vi "Autonomous Independent.vi"   [LabVIEW 2015]
doc: "This VI is called when autonomous begins, and will automatically be terminated when autonomous ends. You can carry out timed or sensor driven robot movement independently without needing to return to the caller."
uses:
  <vilib>/Rock Robotics/WPI/Relay/WPI_RelayValue.ctl
  <vilib>/Rock Robotics/Network Tables/SD Read String.vi
  <vilib>/Rock Robotics/WPI/Utilities/WPI_GetSetVariantRefNum.vi
  Robot Global Data.vi
  <vilib>/Rock Robotics/WPI/RobotDrive/WPI_RobotDriveMecanumDrive_Cartesian.vi
  <vilib>/addons/control/pid/pid.llb/PID (DBL).vi
  <vilib>/Rock Robotics/Network Tables/SD Write Numeric Array.vi
  SimpleGyro/SimpleGyro.lvlib
  <vilib>/addons/control/pid/NI_PID_pid.lvlib
panel:
  # "Be sure to right-click and choose Data Operations>>Make Current Value default if you want to save the array values with the VI"
types:
  T1 = typedef "WPI_RelayValue.ctl" = enum16{"Off", "On", "Forward", "Reverse"}
  T2 = cluster{"proportional gain (Kc)":dbl, "integral time (Ti, min)":dbl, "derivative time (Td, min)":dbl}
  T3 = typedef "SimpleGyro.lvlib/WPI_SimpleGyroDevRef.ctl" = cluster{"DevStatus":errorcluster, "Handle":i32, "SPI Bus":T4, "Device Found":bool, "Sample Rate":dbl}
  T4 = typedef "spi_bus.ctl" = enum16{"SPI On-Board, CS0", "SPI On-Board, CS1", "SPI On-Board, CS2", "SPI On-Board, CS3", "SPI MXP", "Invalid"}
  T5 = typedef "WPI_RobotDriveDevRef.ctl" = cluster{"DevStatus":errorcluster, "Motors[]":T6[], "Square Inputs":bool, "Max Output":dbl}
  T6 = typedef "WPI_MotorControlDeviceRef.ctl" = cluster{"DeviceStatus":errorcluster, "Type":T7, "PWM":cluster{"PWM Channel":T8, "DeadBand":T9}, "CAN":cluster{"Device Number":u8, "Control Mode":T10, "Semaphore":T11, "Max Vout":dbl, "TalonSRX Control Mode":T12}, "Invert":bool, "TransformRef":T13, "InvTransformRef":T13}
  T7 = typedef "WPI_MotorControlType.ctl" = enum16{"PWM", "CAN", "CANTalonSRX"}
  T8 = typedef "FPGA_DIOPWMChannel.ctl" = enum8{"PWM 0", "PWM 1", "PWM 2", "PWM 3", "PWM 4", "PWM 5", "PWM 6", "PWM 7", "PWM 8", "PWM 9", "PWM MXP 0", "PWM MXP 1", "PWM MXP 2", "PWM MXP 3", "PWM MXP 4", "PWM MXP 5", "PWM MXP 6", "PWM MXP 7", "PWM MXP 8", "PWM MXP 9", "Invalid"}
  T9 = typedef "WPI_PWMDeadband.ctl" = cluster{"Name":string, "maxPositivePwm":i32, "minPositivePwm":i32, "centerPwm":i32, "maxNegativePwm":i32, "minNegativePwm":i32, "angularRange":u16}
  T10 = typedef "WPI_CANJaguar_ControlMode.ctl" = enum8{"Percent VBus", "Current", "Speed", "Position", "Voltage"}
  T11 = typedef "Semaphore RefNum" = refnum<k1>
  T12 = typedef "WPI_CANTalonSRX_APIControlMode.ctl" = enum8{"Percent VBus", "Speed", "Position", "Slave", "Unchanged / Invalid"}
  T13 = typedef "WPI_PWMTransform_ConPane.ctl" = refnum<vi>
  T14 = typedef "WPI_EncoderDevRef.ctl" = cluster{"DevStatus":errorcluster, "EncoderIndex":T15, "CounterIndex":T16, "DistancePerCount":dbl, "Decoding Type":T17}
  T15 = typedef "FPGA_EncoderIdx.ctl" = enum8{"Enc 0", "Enc 1", "Enc 2", "Enc 3", "Enc 4", "Enc 5", "Enc 6", "Enc 7", "Invalid"}
  T16 = typedef "FPGA_CounterCtrSystemIndex.ctl" = enum8{"Ctr 0", "Ctr 1", "Ctr 2", "Ctr 3", "Ctr 4", "Ctr 5", "Ctr 6", "Ctr 7", "Invalid"}
  T17 = typedef "WPI_EncoderType.ctl" = enum16{"1x", "2x", "4x"}
  T18 = typedef "WPI_RelayDevRef.ctl" = cluster{"DevStatus":errorcluster, "Relay Channel":T19, "Relay Direction":T20}
  T19 = typedef "FPGA_DIORelayChannel.ctl" = enum8{"Relay 0", "Relay 1", "Relay 2", "Relay 3", "Invalid"}
  T20 = typedef "WPI_RelayDirection.ctl" = enum16{"Both directions", "Forward only", "Reverse only"}
  T21 = cluster{"SimpleGyroDevRef":T3, "RobotDriveDevRef":T5, "EncoderDevRef":T14, "MotorControlDevRef":T6, "RelayDevRef":T18}
  T22 = cluster{"SimpleGyroDevRef":T3, "RobotDriveDevRef":T5, "EncoderDevRef":T14, "MotorControlDevRef":T6, "RelayDevRef":T18, "MotorControlDevRef":T6}
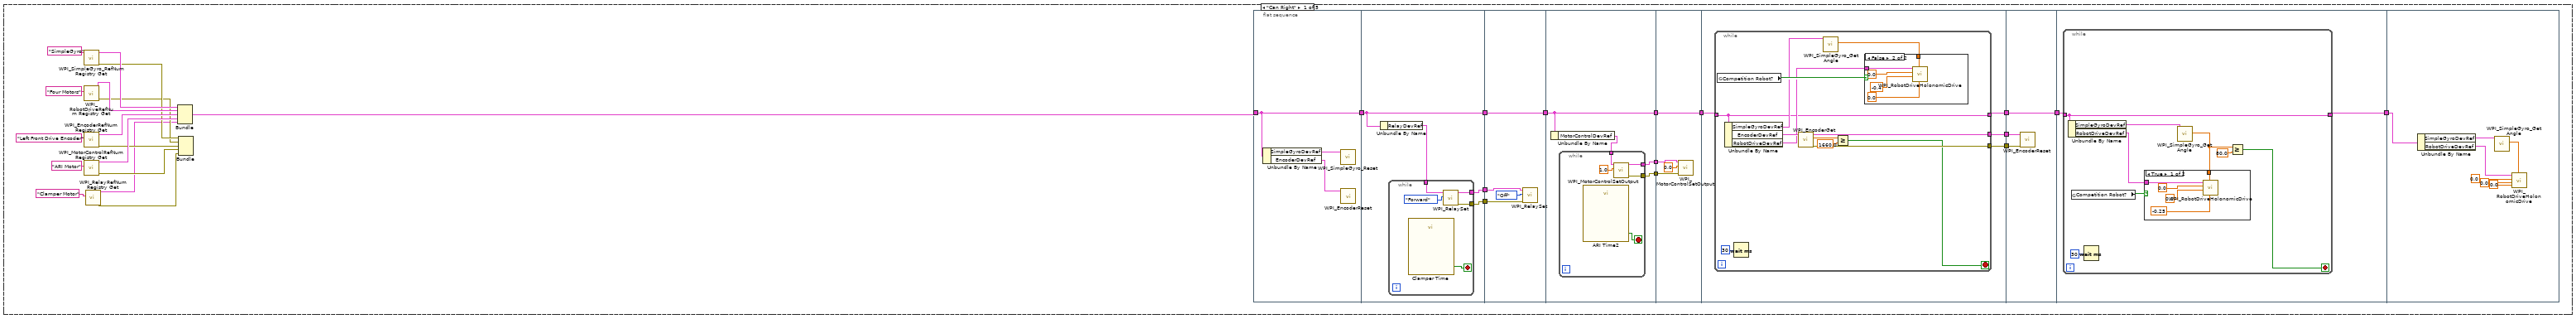
[diagram p2: hidden frame]
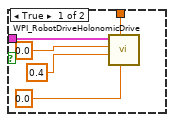
[diagram p3: hidden frame]
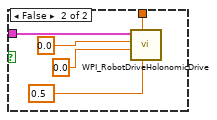
[diagram p4: hidden frame]
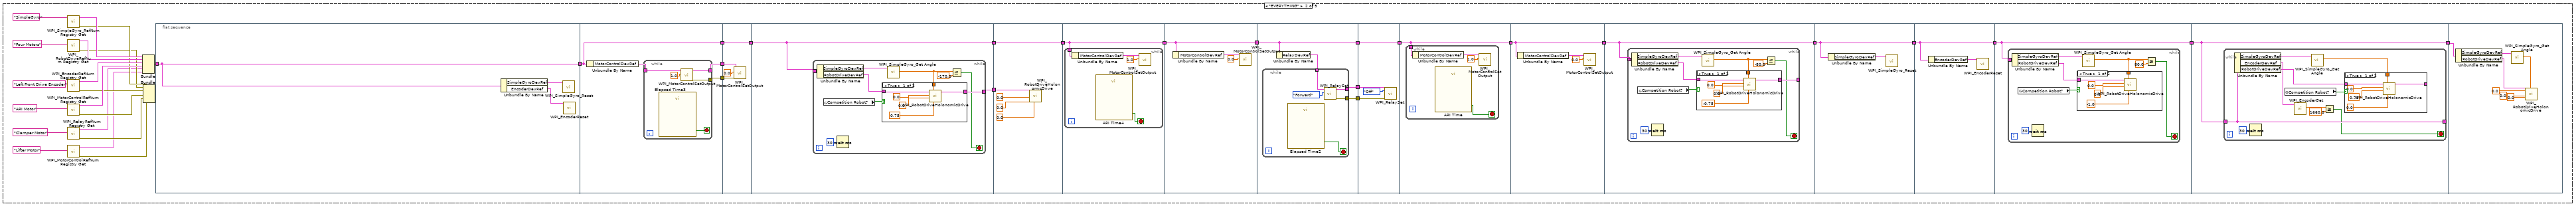
[diagram p5: hidden frame]
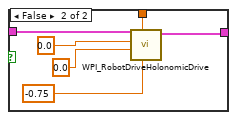
[diagram p6: hidden frame]
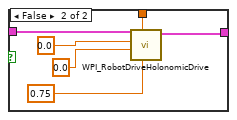
[diagram p7: hidden frame]
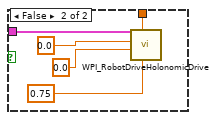
[diagram p8: hidden frame]
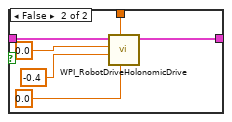
[diagram p9: hidden frame]
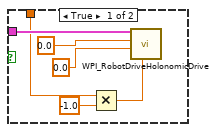
[diagram p10: hidden frame]
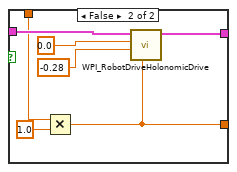
[diagram p11: hidden frame]
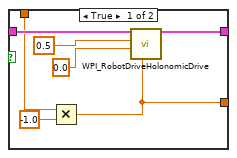
[diagram p12: hidden frame]
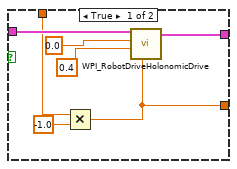
[diagram p13: hidden frame]
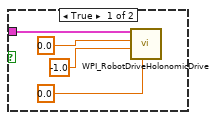
[diagram p14: hidden frame]
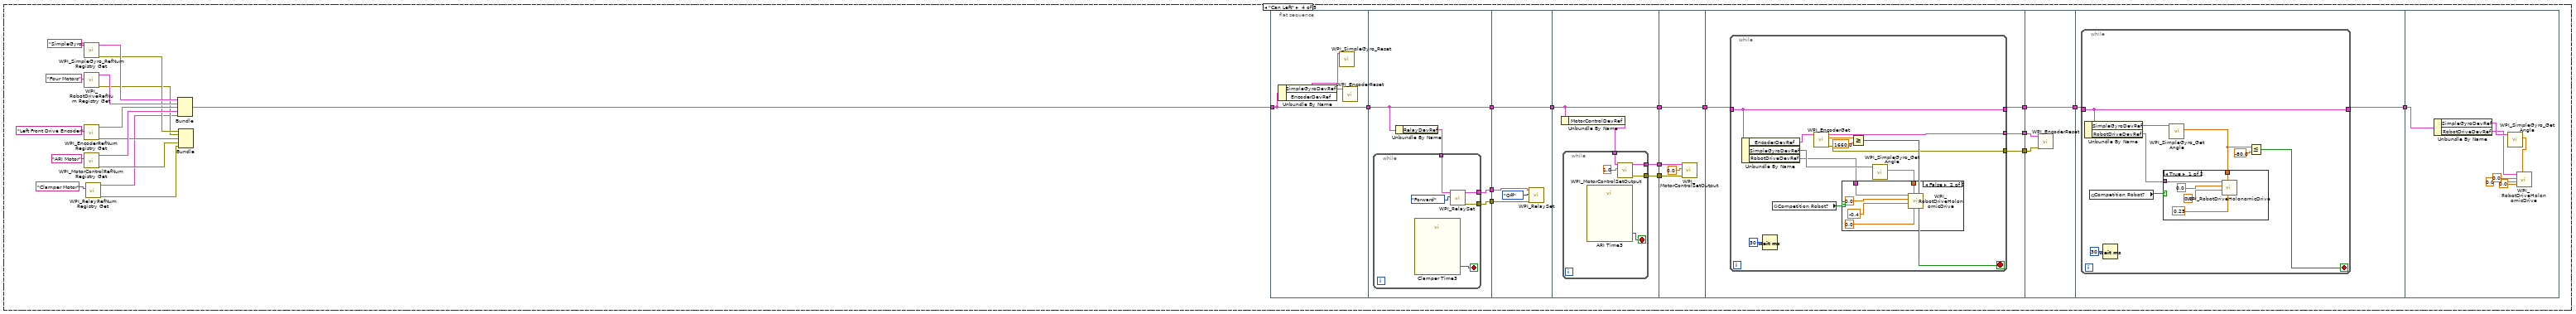
[diagram p15: hidden frame]
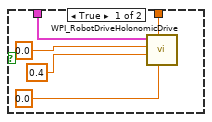
[diagram p16: hidden frame]
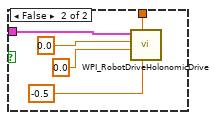
[diagram p17: hidden frame]
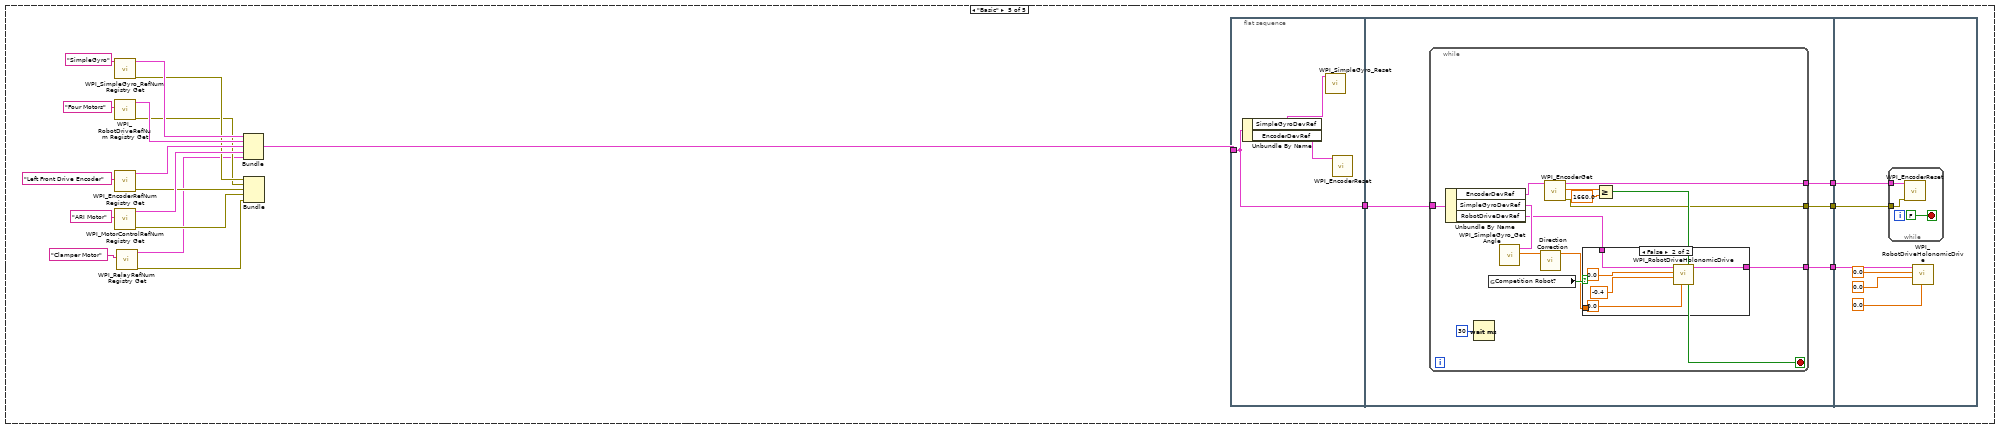
[diagram p18: hidden frame]
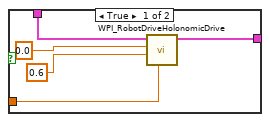
[diagram p19: hidden frame]
diagram:
  # "Every 20ms, report that we are running autonomous\ncode. Loop will abort the same time as the VI."
  n1 = call-poly <vilib>:"SD Read Value.vi"("Name"="AUTO") -> ("String"=w2:string)  [unwired: 8 in, 2 out]
  n2 = case shown="\"Totes Totes\", Default" w2 {
    frame "Can Right" {
      n3 = call "WPI_SimpleGyro_RefNum Registry Get.vi"("refnum name"="SimpleGyro") -> ("error out"=w18:errorcluster, "SimpleGyroDevRef"=w22:T3)  [unwired: 9 in]
      n4 = call <vilib>:"WPI_RobotDriveRefNum Registry Get.vi"("refnum name"="Four Motors") -> ("error out"=w17:errorcluster, "RobotDriveDevRef"=w21:T5)  [unwired: 1 in, 8 out]
      n5 = call <vilib>:"WPI_EncoderRefNum Registry Get.vi"("refnum name"="Left Front Drive Encoder") -> ("error out"=w16:errorcluster, "EncoderDevRef"=w20:T14)  [unwired: 9 in]
      n6 = call <vilib>:"WPI_MotorControlRefNum Registry Get.vi"("refnum name"="ARI Motor") -> ("error out"=w15:errorcluster, "MotorControlDevRef"=w19:T6)  [unwired: 9 in]
      n7 = call <vilib>:"WPI_RelayRefNum Registry Get.vi"("refnum name"="Clamper Motor") -> ("error out"=w10:errorcluster, "RelayDevRef"=w11:T18)  [unwired: 9 in]
      n8 = Bundle("SimpleGyroDevRef"=w22, "RobotDriveDevRef"=w21, "EncoderDevRef"=w20, "MotorControlDevRef"=w19, "RelayDevRef"=w11) -> (w14:T21)  [unwired: 1 in]
      n9 = Bundle("error out"=w18, "error out"=w17, "error out"=w16, "error out"=w15, "error out"=w10) -> ()  [unwired: 1 in, 1 out]
      n10 = flat-sequence {
        tunnel: w14 -> [w33]
        tunnel: [w33] -> w13
        tunnel: [w39] -> w32
        tunnel: [w38] -> w31
        tunnel: w13 -> [w36]
        tunnel: [w36] -> w8
        tunnel: w32 -> [w47]
        tunnel: w31 -> [w46]
        tunnel: [w45] -> w9
        tunnel: w8 -> [w45]
        tunnel: [w52] -> w30
        tunnel: [w51] -> w29
        tunnel: w9 -> [w49]
        tunnel: [w49] -> w6
        tunnel: w30 -> [w60]
        tunnel: w29 -> [w59]
        tunnel: [w58] -> w7
        tunnel: w6 -> [w58]
        tunnel: [w65] -> w28
        tunnel: [w64] -> w27
        tunnel: w7 -> [w63]
        tunnel: [w62] -> w4
        tunnel: w28 -> [w90]
        tunnel: w27 -> [w89]
        tunnel: [w88] -> w5
        tunnel: w4 -> [w88]
        tunnel: w5 -> [w92]
        tunnel: [w91] -> w3
        tunnel: w3 -> [w113]
        frame #0 {
          n11 = Unbundle By Name(w33) -> ("SimpleGyroDevRef"=w35:T3, "EncoderDevRef"=w34:T14)
          n12 = call "WPI_SimpleGyro_Reset.vi"("SimpleGyroDevRef"=w35) -> ()  [unwired: 9 in, 2 out]
          n13 = call <vilib>:"WPI_EncoderReset.vi"("EncoderDevRef"=w34) -> ()  [unwired: 9 in, 2 out]
        }
        frame #1 {
          n14 = Unbundle By Name(w36) -> ("RelayDevRef"=w37:T18)
          n15 = while {
            tunnel: [w43] -> w39
            tunnel: [w42] -> w38
            tunnel: w37 -> [w40]
            stop <- w41 stop-if-true
            n16 = call "Clamper Time"() -> ("Time has Elapsed"=w41:bool)  [unwired: 12 in, 7 out]
            n17 = call <vilib>:"WPI_RelaySet.vi"("RelayValue"=WPI_RelayValue."Forward", "RelayDevRef"=w40) -> ("error out"=w42:errorcluster, "RelayDevRef"=w43:T18)  [unwired: 8 in]
          }
        }
        frame #2 {
          n18 = call <vilib>:"WPI_RelaySet.vi"("error in (no error)"=w46, "RelayValue"=WPI_RelayValue."Off", "RelayDevRef"=w47) -> ()  [unwired: 7 in, 2 out]
        }
        frame #3 {
          n19 = Unbundle By Name(w49) -> ("MotorControlDevRef"=w50:T6)
          n20 = while {
            tunnel: [w55] -> w52
            tunnel: [w54] -> w51
            tunnel: w50 -> [w53]
            stop <- w57 stop-if-true
            n21 = call "ARI Time2"() -> ("Time has Elapsed"=w57:bool)  [unwired: 12 in, 7 out]
            n22 = call <vilib>:"WPI_MotorControlSetOutput.vi"("Output"=1.0, "MotorControlDevRef"=w53) -> ("error out"=w55:errorcluster, "MotorControlDevRef"=w54:T6)  [unwired: 7 in, 1 out]
          }
        }
        frame #4 {
          n23 = call <vilib>:"WPI_MotorControlSetOutput.vi"("error in (no error)"=w60, "Output"=0.0, "MotorControlDevRef"=w59) -> ()  [unwired: 6 in, 3 out]
        }
        frame #5 {
          n24 = while {
            tunnel: [w75] -> w65
            tunnel: [w74] -> w64
            tunnel: w63 -> [w67]
            tunnel: [w67] -> w62
            stop <- w66 stop-if-true
            n25 = global read "Robot Global Data.vi" "Competition Robot?"() -> (w72:bool)
            n26 = Unbundle By Name(w67) -> ("SimpleGyroDevRef"=w70:T3, "EncoderDevRef"=w69:T14, "RobotDriveDevRef"=w68:T5)
            n27 = Wait (ms)(milliseconds to wait=u32 30) -> ()  [unwired: 1 out]
            n28 = call <vilib>:"WPI_EncoderGet.vi"("EncoderDevRef"=w69) -> ("error out"=w74:errorcluster, "Distance"=w77:dbl, "EncoderDevRef"=w75:T14)  [unwired: 5 in, 3 out]
            n29 = call "WPI_SimpleGyro_Get Angle.vi"("SimpleGyroDevRef"=w70) -> ("Angle"=w73:dbl)  [unwired: 8 in, 2 out]
            n30 = Greater Or Equal?(x=w77, y=1660.0) -> (x >= y?=w66:bool)
            n31 = case shown="False" w72 {
              tunnel: w73 -> [w79 w84]
              tunnel: w68 -> [w78 w83]
              frame True {
                n32 = call-poly <vilib>:"WPI_RobotDriveHolonomicDrive.vi"("Rotation"=0.0, "Gyro Angle"=w79, "Y"=0.4 ("X axis value"), "X"=0.0 ("X axis value"), "RobotDriveDevRef"=w78) -> ()  [unwired: 4 in, 3 out]
              }
              frame False {
                n33 = call-poly <vilib>:"WPI_RobotDriveHolonomicDrive.vi"("Rotation"=0.0, "Gyro Angle"=w84, "Y"=-0.4 ("X axis value"), "X"=0.0 ("X axis value"), "RobotDriveDevRef"=w83) -> ()  [unwired: 4 in, 3 out]
              }
            }
          }
        }
        frame #6 {
          n34 = call <vilib>:"WPI_EncoderReset.vi"("error in (no error)"=w89, "EncoderDevRef"=w90) -> ()  [unwired: 8 in, 2 out]
        }
        frame #7 {
          n35 = while {
            tunnel: w92 -> [w93]
            tunnel: [w93] -> w91
            stop <- w97 stop-if-true
            n36 = Unbundle By Name(w93) -> ("SimpleGyroDevRef"=w95:T3, "RobotDriveDevRef"=w94:T5)
            n37 = global read "Robot Global Data.vi" "Competition Robot?"() -> (w99:bool)
            n38 = Wait (ms)(milliseconds to wait=u32 30) -> ()  [unwired: 1 out]
            n39 = call "WPI_SimpleGyro_Get Angle.vi"("SimpleGyroDevRef"=w95) -> ("Angle"=w98:dbl)  [unwired: 8 in, 2 out]
            n40 = case shown="True" w99 {
              tunnel: w98 -> [w102 w107]
              tunnel: w94 -> [w101 w106]
              frame True {
                n41 = call-poly <vilib>:"WPI_RobotDriveHolonomicDrive.vi"("Rotation"=-0.25, "Gyro Angle"=w102, "Y"=0.0 ("X axis value"), "X"=0.0 ("X axis value"), "RobotDriveDevRef"=w101) -> ()  [unwired: 4 in, 3 out]
              }
              frame False {
                n42 = call-poly <vilib>:"WPI_RobotDriveHolonomicDrive.vi"("Rotation"=0.5, "Gyro Angle"=w107, "Y"=0.0 ("X axis value"), "X"=0.0 ("X axis value"), "RobotDriveDevRef"=w106) -> ()  [unwired: 4 in, 3 out]
              }
            }
            n43 = Greater Or Equal?(x=w98, y=80.0) -> (x >= y?=w97:bool)
          }
        }
        frame #8 {
          n44 = Unbundle By Name(w113) -> ("SimpleGyroDevRef"=w111:T3, "RobotDriveDevRef"=w112:T5)
          n45 = call "WPI_SimpleGyro_Get Angle.vi"("SimpleGyroDevRef"=w111) -> ("Angle"=w114:dbl)  [unwired: 8 in, 2 out]
          n46 = call-poly <vilib>:"WPI_RobotDriveHolonomicDrive.vi"("Rotation"=0.0, "Gyro Angle"=w114, "Y"=0.0, "X"=0.0, "RobotDriveDevRef"=w112) -> ()  [unwired: 4 in, 3 out]
        }
      }
    }
    frame "EVERYTHING" {
      n47 = call "WPI_SimpleGyro_RefNum Registry Get.vi"("refnum name"="SimpleGyro") -> ("error out"=w149:errorcluster, "SimpleGyroDevRef"=w153:T3)  [unwired: 9 in]
      n48 = call <vilib>:"WPI_RobotDriveRefNum Registry Get.vi"("refnum name"="Four Motors") -> ("error out"=w148:errorcluster, "RobotDriveDevRef"=w152:T5)  [unwired: 1 in, 8 out]
      n49 = call <vilib>:"WPI_EncoderRefNum Registry Get.vi"("refnum name"="Left Front Drive Encoder") -> ("error out"=w147:errorcluster, "EncoderDevRef"=w151:T14)  [unwired: 9 in]
      n50 = call <vilib>:"WPI_MotorControlRefNum Registry Get.vi"("refnum name"="ARI Motor") -> ("error out"=w146:errorcluster, "MotorControlDevRef"=w150:T6)  [unwired: 9 in]
      n51 = call <vilib>:"WPI_RelayRefNum Registry Get.vi"("refnum name"="Clamper Motor") -> ("error out"=w141:errorcluster, "RelayDevRef"=w142:T18)  [unwired: 9 in]
      n52 = call <vilib>:"WPI_MotorControlRefNum Registry Get.vi"("refnum name"="Lifter Motor") -> ("error out"=w118:errorcluster, "MotorControlDevRef"=w139:T6)  [unwired: 9 in]
      n53 = Bundle("SimpleGyroDevRef"=w153, "RobotDriveDevRef"=w152, "EncoderDevRef"=w151, "MotorControlDevRef"=w150, "RelayDevRef"=w142, "MotorControlDevRef"=w139) -> (w145:T22)  [unwired: 1 in]
      n54 = Bundle("error out"=w149, "error out"=w148, "error out"=w147, "error out"=w146, "error out"=w141, "error out"=w118) -> ()  [unwired: 1 in, 1 out]
      n55 = flat-sequence {
        tunnel: w145 -> [w158]
        tunnel: [w158] -> w144
        tunnel: w144 -> [w163]
        tunnel: [w163] -> w138
        tunnel: [w162] -> w136
        tunnel: [w161] -> w135
        tunnel: w138 -> [w173]
        tunnel: [w173] -> w137
        tunnel: w136 -> [w172]
        tunnel: w135 -> [w171]
        tunnel: w137 -> [w175]
        tunnel: [w175] -> w134
        tunnel: [w174] -> w133
        tunnel: w134 -> [w201]
        tunnel: [w201] -> w127
        tunnel: w133 -> [w200]
        tunnel: w127 -> [w202]
        tunnel: [w202] -> w126
        tunnel: w126 -> [w207]
        tunnel: [w207] -> w125
        tunnel: w125 -> [w212]
        tunnel: [w212] -> w132
        tunnel: [w211] -> w131
        tunnel: [w210] -> w130
        tunnel: w132 -> [w222]
        tunnel: [w222] -> w129
        tunnel: w131 -> [w220]
        tunnel: w130 -> [w219]
        tunnel: w129 -> [w223]
        tunnel: [w223] -> w128
        tunnel: w128 -> [w228]
        tunnel: [w228] -> w124
        tunnel: w124 -> [w231]
        tunnel: [w231] -> w123
        tunnel: w123 -> [w254]
        tunnel: [w254] -> w122
        tunnel: w122 -> [w256]
        tunnel: [w256] -> w121
        tunnel: w121 -> [w257]
        tunnel: [w257] -> w120
        tunnel: w120 -> [w276]
        tunnel: [w276] -> w119
        tunnel: w119 -> [w299]
        frame #0 {
          n56 = Unbundle By Name(w158) -> ("SimpleGyroDevRef"=w160:T3, "EncoderDevRef"=w159:T14)
          n57 = call "WPI_SimpleGyro_Reset.vi"("SimpleGyroDevRef"=w160) -> ()  [unwired: 9 in, 2 out]
          n58 = call <vilib>:"WPI_EncoderReset.vi"("EncoderDevRef"=w159) -> ()  [unwired: 9 in, 2 out]
        }
        frame #1 {
          n59 = Unbundle By Name(w163) -> ("MotorControlDevRef"=w164:T6)
          n60 = while {
            tunnel: w164 -> [w168]
            tunnel: [w166] -> w162
            tunnel: [w165] -> w161
            stop <- w169 stop-if-true
            n61 = call "Elapsed Time3"() -> ("Time has Elapsed"=w169:bool)  [unwired: 12 in, 7 out]
            n62 = call <vilib>:"WPI_MotorControlSetOutput.vi"("Output"=1.0, "MotorControlDevRef"=w168) -> ("error out"=w165:errorcluster, "MotorControlDevRef"=w166:T6)  [unwired: 7 in, 1 out]
          }
        }
        frame #2 {
          n63 = call <vilib>:"WPI_MotorControlSetOutput.vi"("error in (no error)"=w171, "Output"=0.0, "MotorControlDevRef"=w172) -> ()  [unwired: 6 in, 3 out]
        }
        frame #3 {
          n64 = while {
            tunnel: w175 -> [w179]
            tunnel: [w177] -> w174
            stop <- w176 stop-if-true
            n65 = Unbundle By Name(w179) -> ("SimpleGyroDevRef"=w178:T3, "RobotDriveDevRef"=w180:T5)
            n66 = global read "Robot Global Data.vi" "Competition Robot?"() -> (w183:bool)
            n67 = Wait (ms)(milliseconds to wait=u32 30) -> ()  [unwired: 1 out]
            n68 = call "WPI_SimpleGyro_Get Angle.vi"("SimpleGyroDevRef"=w178) -> ("Angle"=w182:dbl)  [unwired: 8 in, 2 out]
            n69 = case shown="True" w183 {
              tunnel: w182 -> [w187 w193]
              tunnel: w180 -> [w186 w191]
              tunnel: [w185 w192] -> w177
              frame True {
                n70 = call-poly <vilib>:"WPI_RobotDriveHolonomicDrive.vi"("Rotation"=0.75, "Gyro Angle"=w187, "Y"=0.0 ("X axis value"), "X"=0.0 ("X axis value"), "RobotDriveDevRef"=w186) -> ("RobotDriveDevRef"=w185:T5)  [unwired: 4 in, 2 out]
              }
              frame False {
                n71 = call-poly <vilib>:"WPI_RobotDriveHolonomicDrive.vi"("Rotation"=-0.75, "Gyro Angle"=w193, "Y"=0.0 ("X axis value"), "X"=0.0 ("X axis value"), "RobotDriveDevRef"=w191) -> ("RobotDriveDevRef"=w192:T5)  [unwired: 4 in, 2 out]
              }
            }
            n72 = Less Or Equal?(x=w182, y=-170.0) -> (x <= y?=w176:bool)
          }
        }
        frame #4 {
          n73 = call-poly <vilib>:"WPI_RobotDriveHolonomicDrive.vi"("Rotation"=0.0, "Y"=0.0, "X"=0.0, "RobotDriveDevRef"=w200) -> ()  [unwired: 5 in, 3 out]
        }
        frame #5 {
          n74 = while {
            tunnel: w202 -> [w203]
            stop <- w206 stop-if-true
            n75 = Unbundle By Name(w203) -> ("MotorControlDevRef"=w205:T6)
            n76 = call "ARI Time4"() -> ("Time has Elapsed"=w206:bool)  [unwired: 12 in, 7 out]
            n77 = call <vilib>:"WPI_MotorControlSetOutput.vi"("Output"=1.0, "MotorControlDevRef"=w205) -> ()  [unwired: 7 in, 3 out]
          }
        }
        frame #6 {
          n78 = Unbundle By Name(w207) -> ("MotorControlDevRef"=w208:T6)
          n79 = call <vilib>:"WPI_MotorControlSetOutput.vi"("Output"=0.0, "MotorControlDevRef"=w208) -> ()  [unwired: 7 in, 3 out]
        }
        frame #7 {
          n80 = Unbundle By Name(w212) -> ("RelayDevRef"=w213:T18)
          n81 = while {
            tunnel: [w217] -> w211
            tunnel: [w216] -> w210
            tunnel: w213 -> [w214]
            stop <- w215 stop-if-true
            n82 = call "Elapsed Time2"() -> ("Time has Elapsed"=w215:bool)  [unwired: 12 in, 7 out]
            n83 = call <vilib>:"WPI_RelaySet.vi"("RelayValue"=WPI_RelayValue."Forward", "RelayDevRef"=w214) -> ("error out"=w216:errorcluster, "RelayDevRef"=w217:T18)  [unwired: 8 in]
          }
        }
        frame #8 {
          n84 = call <vilib>:"WPI_RelaySet.vi"("error in (no error)"=w219, "RelayValue"=WPI_RelayValue."Off", "RelayDevRef"=w220) -> ()  [unwired: 7 in, 2 out]
        }
        frame #9 {
          n85 = while {
            tunnel: w223 -> [w224]
            stop <- w227 stop-if-true
            n86 = Unbundle By Name(w224) -> ("MotorControlDevRef"=w226:T6)
            n87 = call "ARI Time"() -> ("Time has Elapsed"=w227:bool)  [unwired: 12 in, 7 out]
            n88 = call <vilib>:"WPI_MotorControlSetOutput.vi"("Output"=1.0, "MotorControlDevRef"=w226) -> ()  [unwired: 7 in, 3 out]
          }
        }
        frame #10 {
          n89 = Unbundle By Name(w228) -> ("MotorControlDevRef"=w229:T6)
          n90 = call <vilib>:"WPI_MotorControlSetOutput.vi"("Output"=0.0, "MotorControlDevRef"=w229) -> ()  [unwired: 7 in, 3 out]
        }
        frame #11 {
          n91 = while {
            tunnel: w231 -> [w235]
            tunnel: [w233] -> _
            stop <- w232 stop-if-true
            n92 = Unbundle By Name(w235) -> ("SimpleGyroDevRef"=w234:T3, "RobotDriveDevRef"=w236:T5)
            n93 = global read "Robot Global Data.vi" "Competition Robot?"() -> (w239:bool)
            n94 = Wait (ms)(milliseconds to wait=u32 30) -> ()  [unwired: 1 out]
            n95 = call "WPI_SimpleGyro_Get Angle.vi"("SimpleGyroDevRef"=w234) -> ("Angle"=w238:dbl)  [unwired: 8 in, 2 out]
            n96 = case shown="True" w239 {
              tunnel: w238 -> [w243 w249]
              tunnel: w236 -> [w242 w247]
              tunnel: [w241 w248] -> w233
              frame True {
                n97 = call-poly <vilib>:"WPI_RobotDriveHolonomicDrive.vi"("Rotation"=-0.75, "Gyro Angle"=w243, "Y"=0.0 ("X axis value"), "X"=0.0 ("X axis value"), "RobotDriveDevRef"=w242) -> ("RobotDriveDevRef"=w241:T5)  [unwired: 4 in, 2 out]
              }
              frame False {
                n98 = call-poly <vilib>:"WPI_RobotDriveHolonomicDrive.vi"("Rotation"=0.75, "Gyro Angle"=w249, "Y"=0.0 ("X axis value"), "X"=0.0 ("X axis value"), "RobotDriveDevRef"=w247) -> ("RobotDriveDevRef"=w248:T5)  [unwired: 4 in, 2 out]
              }
            }
            n99 = Less Or Equal?(x=w238, y=-80.0) -> (x <= y?=w232:bool)
          }
        }
        frame #12 {
          n100 = Unbundle By Name(w254) -> ("SimpleGyroDevRef"=w253:T3)
          n101 = call "WPI_SimpleGyro_Reset.vi"("SimpleGyroDevRef"=w253) -> ()  [unwired: 9 in, 2 out]
        }
        frame #13 {
          n102 = Unbundle By Name(w256) -> ("EncoderDevRef"=w255:T14)
          n103 = call <vilib>:"WPI_EncoderReset.vi"("EncoderDevRef"=w255) -> ()  [unwired: 9 in, 2 out]
        }
        frame #14 {
          n104 = while {
            tunnel: w257 -> [w259]
            stop <- w260 stop-if-true
            n105 = Unbundle By Name(w259) -> ("SimpleGyroDevRef"=w258:T3, "RobotDriveDevRef"=w261:T5)
            n106 = global read "Robot Global Data.vi" "Competition Robot?"() -> (w264:bool)
            n107 = Wait (ms)(milliseconds to wait=u32 30) -> ()  [unwired: 1 out]
            n108 = call "WPI_SimpleGyro_Get Angle.vi"("SimpleGyroDevRef"=w258) -> ("Angle"=w263:dbl)  [unwired: 8 in, 2 out]
            n109 = case shown="True" w264 {
              tunnel: w263 -> [w267 w272]
              tunnel: w261 -> [w266 w271]
              frame True {
                n110 = call-poly <vilib>:"WPI_RobotDriveHolonomicDrive.vi"("Rotation"=-1.0, "Gyro Angle"=w267, "Y"=0.0 ("X axis value"), "X"=0.0 ("X axis value"), "RobotDriveDevRef"=w266) -> ()  [unwired: 4 in, 3 out]
              }
              frame False {
                n111 = call-poly <vilib>:"WPI_RobotDriveHolonomicDrive.vi"("Rotation"=0.75, "Gyro Angle"=w272, "Y"=0.0 ("X axis value"), "X"=0.0 ("X axis value"), "RobotDriveDevRef"=w271) -> ()  [unwired: 4 in, 3 out]
              }
            }
            n112 = Greater Or Equal?(x=w263, y=80.0) -> (x >= y?=w260:bool)
          }
        }
        frame #15 {
          n113 = while {
            tunnel: w276 -> [w281]
            tunnel: [w281] -> _
            stop <- w280 stop-if-true
            n114 = Unbundle By Name(w281) -> ("SimpleGyroDevRef"=w278:T3, "EncoderDevRef"=w277:T14, "RobotDriveDevRef"=w279:T5)
            n115 = Wait (ms)(milliseconds to wait=u32 30) -> ()  [unwired: 1 out]
            n116 = global read "Robot Global Data.vi" "Competition Robot?"() -> (w283:bool)
            n117 = call <vilib>:"WPI_EncoderGet.vi"("EncoderDevRef"=w277) -> ("Distance"=w286:dbl)  [unwired: 5 in, 5 out]
            n118 = call "WPI_SimpleGyro_Get Angle.vi"("SimpleGyroDevRef"=w278) -> ("Angle"=w284:dbl)  [unwired: 8 in, 2 out]
            n119 = Greater Or Equal?(x=w286, y=1660.0) -> (x >= y?=w280:bool)
            n120 = case shown="True" w283 {
              tunnel: w284 -> [w289 w295]
              tunnel: w279 -> [w287 w294]
              tunnel: [w288 w293] -> _
              frame True {
                n121 = call-poly <vilib>:"WPI_RobotDriveHolonomicDrive.vi"("Rotation"=0.0, "Gyro Angle"=w289, "Y"=0.75 ("X axis value"), "X"=0.0 ("X axis value"), "RobotDriveDevRef"=w287) -> ("RobotDriveDevRef"=w288:T5)  [unwired: 4 in, 2 out]
              }
              frame False {
                n122 = call-poly <vilib>:"WPI_RobotDriveHolonomicDrive.vi"("Rotation"=0.0, "Gyro Angle"=w295, "Y"=-0.4 ("X axis value"), "X"=0.0 ("X axis value"), "RobotDriveDevRef"=w294) -> ("RobotDriveDevRef"=w293:T5)  [unwired: 4 in, 2 out]
              }
            }
          }
        }
        frame #16 {
          n123 = Unbundle By Name(w299) -> ("SimpleGyroDevRef"=w300:T3, "RobotDriveDevRef"=w301:T5)
          n124 = call "WPI_SimpleGyro_Get Angle.vi"("SimpleGyroDevRef"=w300) -> ("Angle"=w302:dbl)  [unwired: 8 in, 2 out]
          n125 = call-poly <vilib>:"WPI_RobotDriveHolonomicDrive.vi"("Rotation"=0.0, "Gyro Angle"=w302, "Y"=0.0, "X"=0.0, "RobotDriveDevRef"=w301) -> ()  [unwired: 4 in, 3 out]
        }
      }
    }
    frame "Totes Totes", Default {
      n126 = call "WPI_SimpleGyro_RefNum Registry Get.vi"("refnum name"="SimpleGyro") -> ("error out"=w350:errorcluster, "SimpleGyroDevRef"=w354:T3)  [unwired: 9 in]
      n127 = call <vilib>:"WPI_RobotDriveRefNum Registry Get.vi"("refnum name"="Four Motors") -> ("error out"=w349:errorcluster, "RobotDriveDevRef"=w353:T5)  [unwired: 1 in, 8 out]
      n128 = call <vilib>:"WPI_EncoderRefNum Registry Get.vi"("refnum name"="Left Front Drive Encoder") -> ("error out"=w348:errorcluster, "EncoderDevRef"=w352:T14)  [unwired: 9 in]
      n129 = call <vilib>:"WPI_MotorControlRefNum Registry Get.vi"("refnum name"="ARI Motor") -> ("error out"=w347:errorcluster, "MotorControlDevRef"=w351:T6)  [unwired: 9 in]
      n130 = call <vilib>:"WPI_RelayRefNum Registry Get.vi"("refnum name"="Clamper Motor") -> ("error out"=w344:errorcluster, "RelayDevRef"=w345:T18)  [unwired: 9 in]
      n131 = call <vilib>:"WPI_MotorControlRefNum Registry Get.vi"("refnum name"="Lifter Motor") -> ("error out"=w340:errorcluster, "MotorControlDevRef"=w341:T6)  [unwired: 9 in]
      n132 = Bundle("SimpleGyroDevRef"=w354, "RobotDriveDevRef"=w353, "EncoderDevRef"=w352, "MotorControlDevRef"=w351, "RelayDevRef"=w345, "MotorControlDevRef"=w341) -> (w313:T22)  [unwired: 1 in]
      n133 = Bundle("error out"=w350, "error out"=w349, "error out"=w348, "error out"=w347, "error out"=w344, "error out"=w340) -> ()  [unwired: 1 in, 1 out]
      n134 = flat-sequence {
        tunnel: w313 -> [w359]
        tunnel: [w359] -> w343
        tunnel: w343 -> [w364]
        tunnel: [w364] -> w336
        tunnel: [w363] -> w334
        tunnel: [w362] -> w333
        tunnel: w336 -> [w390]
        tunnel: [w390] -> w335
        tunnel: w334 -> [w389]
        tunnel: w333 -> [w387]
        tunnel: w335 -> [w393]
        tunnel: [w393] -> w339
        tunnel: [w391] -> w338
        tunnel: w339 -> [w400]
        tunnel: w338 -> [w399]
        tunnel: [w400] -> w337
        tunnel: w337 -> [w403]
        tunnel: [w403] -> w318
        tunnel: w318 -> [w425]
        tunnel: [w425] -> w317
        tunnel: w317 -> [w430]
        tunnel: [w430] -> w320
        tunnel: [w429] -> w319
        tunnel: [w427] -> w312
        tunnel: [w426] -> w311
        tunnel: w320 -> [w466]
        tunnel: [w466] -> w315
        tunnel: w319 -> [w465]
        tunnel: w312 -> [w464]
        tunnel: w311 -> [w462]
        tunnel: w315 -> [w467]
        tunnel: [w467] -> w314
        tunnel: w314 -> [w471]
        tunnel: [w471] -> w332
        tunnel: [w469] -> w331
        tunnel: w332 -> [w476]
        tunnel: w331 -> [w478]
        tunnel: [w476] -> w316
        tunnel: w316 -> [w483]
        tunnel: [w483] -> w330
        tunnel: [w482] -> w329
        tunnel: [w480] -> w310
        tunnel: [w479] -> w309
        tunnel: w330 -> [w517]
        tunnel: w329 -> [w516]
        tunnel: [w517] -> w328
        tunnel: w310 -> [w515]
        tunnel: w309 -> [w514]
        tunnel: w328 -> [w521]
        tunnel: [w521] -> w327
        tunnel: [w522] -> w326
        tunnel: [w519] -> w308
        tunnel: [w518] -> w307
        tunnel: w327 -> [w552]
        tunnel: w326 -> [w556]
        tunnel: w308 -> [w554]
        tunnel: w307 -> [w553]
        tunnel: [w552] -> w306
        tunnel: w306 -> [w557]
        tunnel: [w557] -> w325
        tunnel: w325 -> [w578]
        tunnel: [w578] -> w324
        tunnel: [w577] -> w323
        tunnel: [w576] -> w322
        tunnel: w324 -> [w604]
        tunnel: w323 -> [w603]
        tunnel: w322 -> [w602]
        tunnel: [w604] -> w321
        tunnel: [w605] -> _
        tunnel: w321 -> [w605]
        frame #0 {
          n135 = Unbundle By Name(w359) -> ("SimpleGyroDevRef"=w360:T3, "EncoderDevRef"=w361:T14)
          n136 = call "WPI_SimpleGyro_Reset.vi"("SimpleGyroDevRef"=w360) -> ()  [unwired: 9 in, 2 out]
          n137 = call <vilib>:"WPI_EncoderReset.vi"("EncoderDevRef"=w361) -> ()  [unwired: 9 in, 2 out]
        }
        frame #1 {
          # "Simultaneously lowers ARI"
          # "Picks up tote"
          n138 = while {
            tunnel: w364 -> [w374]
            tunnel: [w366] -> w363
            tunnel: [w365] -> w362
            stop <- w371 stop-if-true
            n139 = Unbundle By Name(w374) -> ("MotorControlDevRef"=w373:T6, "MotorControlDevRef"=w372:T6)
            n140 = while {
              tunnel: w373 -> [w385]
              tunnel: [w383] -> w369
              tunnel: [w382] -> w366
              stop <- w383 stop-if-true
              n141 = call "Elapsed Time"() -> ("Time has Elapsed"=w383:bool)  [unwired: 12 in, 7 out]
              n142 = call <vilib>:"WPI_MotorControlSetOutput.vi"("Output"=1.0, "MotorControlDevRef"=w385) -> ("MotorControlDevRef"=w382:T6)  [unwired: 7 in, 2 out]
            }
            n143 = global read "Robot Global Data.vi" "Competition Robot?"() -> (w370:bool)
            n144 = while {
              tunnel: w372 -> [w381]
              tunnel: w370 -> [w379]
              tunnel: [w376] -> w368
              tunnel: [w375] -> w365
              stop <- w376 stop-if-true
              n145 = Select(t=-1.0, s=w379, f=0.0) -> (s? t:f=w380:dbl)
              n146 = call "ARI Time5"() -> ("Time has Elapsed"=w376:bool)  [unwired: 12 in, 7 out]
              n147 = call <vilib>:"WPI_MotorControlSetOutput.vi"("Output"=w380, "MotorControlDevRef"=w381) -> ("MotorControlDevRef"=w375:T6)  [unwired: 7 in, 2 out]
            }
            n148 = And(x=w368, y=w369) -> (x .and. y?=w367:bool)
            n149 = Select(t=w367, s=w370, f=w369) -> (s? t:f=w371:bool)
          }
        }
        frame #2 {
          n150 = call <vilib>:"WPI_MotorControlSetOutput.vi"("Output"=0.0, "MotorControlDevRef"=w389) -> ()  [unwired: 7 in, 3 out]
          n151 = call <vilib>:"WPI_MotorControlSetOutput.vi"("Output"=0.0, "MotorControlDevRef"=w387) -> ()  [unwired: 7 in, 3 out]
        }
        frame #3 {
          # "Clamper"
          n152 = Unbundle By Name(w393) -> ("RelayDevRef"=w392:T18)
          n153 = while {
            tunnel: [w396] -> _
            tunnel: w392 -> [w395]
            tunnel: [w394] -> w391
            stop <- w396 stop-if-true
            n154 = call "Elapsed Time4"() -> ("Time has Elapsed"=w396:bool)  [unwired: 12 in, 7 out]
            n155 = call <vilib>:"WPI_RelaySet.vi"("RelayValue"=WPI_RelayValue."Forward", "RelayDevRef"=w395) -> ("RelayDevRef"=w394:T18)  [unwired: 8 in, 1 out]
          }
        }
        frame #4 {
          n156 = call <vilib>:"WPI_RelaySet.vi"("RelayValue"=WPI_RelayValue."Off", "RelayDevRef"=w399) -> ()  [unwired: 8 in, 2 out]
        }
        frame #5 {
          # "Turns 180 degrees while carrying tote"
          n157 = Unbundle By Name(w403) -> ("SimpleGyroDevRef"=w402:T3, "RobotDriveDevRef"=w401:T5)
          n158 = while {
            tunnel: w402 -> [w410]
            tunnel: w401 -> [w409]
            stop <- w411 stop-if-true
            n159 = global read "Robot Global Data.vi" "Competition Robot?"() -> (w412:bool)
            n160 = call "WPI_SimpleGyro_Get Angle.vi"("SimpleGyroDevRef"=w410) -> ("Angle"=w404:dbl)  [unwired: 8 in, 2 out]
            n161 = call-poly <vilib>:"PID.vi"("output range"=cluster{"output high":dbl, "output low":dbl} {"output high"=0.4, "output low"=-0.4}, "PID gains"=T2 {"proportional gain (Kc)"=1.0, "integral time (Ti, min)"=0.001, "derivative time (Td, min)"=0.0}, "process variable"=w404, "setpoint"=180.0) -> ("output"=w405:dbl)  [unwired: 6 in, 1 out]
            n162 = case shown="False" w412 {
              tunnel: w409 -> [w417 w421]
              tunnel: w405 -> [w416 w420]
              frame True {
                n163 = Multiply(x=w416, y=-1.0) -> (x*y=w414:dbl)
                n164 = call-poly <vilib>:"WPI_RobotDriveHolonomicDrive.vi"("Rotation"=w414, "Y"=0.0 ("X axis value"), "X"=0.0 ("X axis value"), "RobotDriveDevRef"=w417) -> ()  [unwired: 5 in, 3 out]
              }
              frame False {
                n165 = call-poly <vilib>:"WPI_RobotDriveHolonomicDrive.vi"("Rotation"=w420, "Y"=0.0 ("X axis value"), "X"=0.0 ("X axis value"), "RobotDriveDevRef"=w421) -> ()  [unwired: 5 in, 3 out]
              }
            }
            n166 = Greater Or Equal?(x=w404, y=175.0) -> (x >= y?=w411:bool)
          }
        }
        frame #6 {
          n167 = Unbundle By Name(w425) -> ("EncoderDevRef"=w424:T14)
          n168 = call <vilib>:"WPI_EncoderReset.vi"("EncoderDevRef"=w424) -> ()  [unwired: 9 in, 2 out]
        }
        frame #7 {
          # "Drive Forward to pick up tote #2"
          n169 = Unbundle By Name(w430) -> ("SimpleGyroDevRef"=w428:T3, "RobotDriveDevRef"=w432:T5, "EncoderDevRef"=w431:T14)
          n170 = while {
            tunnel: w432 -> [w443]
            tunnel: w431 -> [w442]
            tunnel: [w441] -> w429
            tunnel: w428 -> [w438]
            tunnel: [w434] -> w427
            tunnel: [w433] -> w426
            stop <- w444 stop-if-true
            n171 = global read "Robot Global Data.vi" "Competition Robot?"() -> (w447:bool)
            n172 = call "WPI_SimpleGyro_Get Angle.vi"("SimpleGyroDevRef"=w438) -> ("Angle"=w437:dbl)  [unwired: 8 in, 2 out]
            n173 = call <vilib>:"WPI_EncoderGet.vi"("EncoderDevRef"=w442) -> ("Distance"=w446:dbl, "EncoderDevRef"=w441:T14)  [unwired: 5 in, 4 out]
            n174 = call-poly <vilib>:"PID.vi"("output range"=cluster{"output high":dbl, "output low":dbl} {"output high"=0.2, "output low"=-0.2}, "PID gains"=T2 {"proportional gain (Kc)"=1.0, "integral time (Ti, min)"=0.03, "derivative time (Td, min)"=0.008}, "process variable"=w437, "setpoint"=180.0) -> ("output"=w435:dbl)  [unwired: 6 in, 1 out]
            n175 = case shown="True" w447 {
              tunnel: w443 -> [w452 w459]
              tunnel: w435 -> [w450 w458]
              tunnel: [w449 w456] -> w434
              tunnel: [w448 w455] -> w433
              frame True {
                n176 = Multiply(x=w450, y=-1.0) -> (x*y=w448:dbl)
                n177 = call-poly <vilib>:"WPI_RobotDriveHolonomicDrive.vi"("Rotation"=w448, "Y"=0.28 ("X axis value"), "X"=0.0 ("X axis value"), "RobotDriveDevRef"=w452) -> ("RobotDriveDevRef"=w449:T5)  [unwired: 5 in, 2 out]
              }
              frame False {
                n178 = Multiply(x=w458, y=1.0) -> (x*y=w455:dbl)
                n179 = call-poly <vilib>:"WPI_RobotDriveHolonomicDrive.vi"("Rotation"=w455, "Y"=-0.28 ("X axis value"), "X"=0.0 ("X axis value"), "RobotDriveDevRef"=w459) -> ("RobotDriveDevRef"=w456:T5)  [unwired: 5 in, 2 out]
              }
            }
            n180 = Greater Or Equal?(x=w446, y=330.0) -> (x >= y?=w444:bool)
          }
        }
        frame #8 {
          w463 = 0.0 ("X")
          n181 = call <vilib>:"WPI_EncoderReset.vi"("EncoderDevRef"=w465) -> ()  [unwired: 9 in, 2 out]
          n182 = call-poly <vilib>:"WPI_RobotDriveHolonomicDrive.vi"("Rotation"=w462, "Y"=w463, "X"=w463, "RobotDriveDevRef"=w464) -> ()  [unwired: 5 in, 3 out]
        }
        frame #9 {
          n183 = while {
            stop <- w468 stop-if-true
            n184 = call "Elapsed Time9"() -> ("Time has Elapsed"=w468:bool)  [unwired: 12 in, 7 out]
          }
        }
        frame #10 {
          # "Picks up second tote"
          n185 = Unbundle By Name(w471) -> ("MotorControlDevRef"=w470:T6)
          n186 = while {
            tunnel: w470 -> [w473]
            tunnel: [w472] -> w469
            stop <- w474 stop-if-true
            n187 = call "Elapsed Time5"() -> ("Time has Elapsed"=w474:bool)  [unwired: 12 in, 7 out]
            n188 = call <vilib>:"WPI_MotorControlSetOutput.vi"("Output"=1.0, "MotorControlDevRef"=w473) -> ("MotorControlDevRef"=w472:T6)  [unwired: 7 in, 2 out]
          }
        }
        frame #11 {
          n189 = call <vilib>:"WPI_MotorControlSetOutput.vi"("Output"=0.0, "MotorControlDevRef"=w478) -> ()  [unwired: 7 in, 3 out]
        }
        frame #12 {
          # "Strafe Left Around Tote #2"
          n190 = Unbundle By Name(w483) -> ("SimpleGyroDevRef"=w481:T3, "RobotDriveDevRef"=w485:T5, "EncoderDevRef"=w484:T14)
          n191 = while {
            tunnel: w485 -> [w496]
            tunnel: w484 -> [w495]
            tunnel: [w494] -> w482
            tunnel: w481 -> [w490]
            tunnel: [w487] -> w480
            tunnel: [w486] -> w479
            stop <- w497 stop-if-true
            n192 = global read "Robot Global Data.vi" "Competition Robot?"() -> (w500:bool)
            n193 = call "WPI_SimpleGyro_Get Angle.vi"("SimpleGyroDevRef"=w490) -> ("Angle"=w489:dbl)  [unwired: 8 in, 2 out]
            n194 = call <vilib>:"WPI_EncoderGet.vi"("EncoderDevRef"=w495) -> ("Distance"=w499:dbl, "EncoderDevRef"=w494:T14)  [unwired: 5 in, 4 out]
            n195 = call-poly <vilib>:"PID.vi"("output range"=cluster{"output high":dbl, "output low":dbl} {"output high"=0.2, "output low"=-0.2}, "PID gains"=T2 {"proportional gain (Kc)"=1.0, "integral time (Ti, min)"=0.035, "derivative time (Td, min)"=0.005}, "process variable"=w489, "setpoint"=180.0) -> ("output"=w488:dbl)  [unwired: 6 in, 1 out]
            n196 = case shown="False" w500 {
              tunnel: w496 -> [w505 w510]
              tunnel: w488 -> [w504 w508]
              tunnel: [w502 w509] -> w487
              tunnel: [w501 w508] -> w486
              frame True {
                n197 = Multiply(x=w504, y=-1.0) -> (x*y=w501:dbl)
                n198 = call-poly <vilib>:"WPI_RobotDriveHolonomicDrive.vi"("Rotation"=w501, "Y"=0.0 ("X axis value"), "X"=0.5 ("X axis value"), "RobotDriveDevRef"=w505) -> ("RobotDriveDevRef"=w502:T5)  [unwired: 5 in, 2 out]
              }
              frame False {
                n199 = call-poly <vilib>:"WPI_RobotDriveHolonomicDrive.vi"("Rotation"=w508, "Y"=0.0 ("X axis value"), "X"=-0.5 ("X axis value"), "RobotDriveDevRef"=w510) -> ("RobotDriveDevRef"=w509:T5)  [unwired: 5 in, 2 out]
              }
            }
            n200 = Less Or Equal?(x=w499, y=-560.0) -> (x <= y?=w497:bool)
          }
        }
        frame #13 {
          w513 = 0.0 ("X")
          # "Stop Motors"
          n201 = call <vilib>:"WPI_EncoderReset.vi"("EncoderDevRef"=w516) -> ()  [unwired: 9 in, 2 out]
          n202 = call-poly <vilib>:"WPI_RobotDriveHolonomicDrive.vi"("Rotation"=w514, "Y"=w513, "X"=w513, "RobotDriveDevRef"=w515) -> ()  [unwired: 5 in, 3 out]
        }
        frame #14 {
          # "Drive Forward to Tote #3"
          n203 = Unbundle By Name(w521) -> ("SimpleGyroDevRef"=w520:T3, "RobotDriveDevRef"=w524:T5, "EncoderDevRef"=w523:T14)
          n204 = while {
            tunnel: w524 -> [w535]
            tunnel: w523 -> [w534]
            tunnel: [w533] -> w522
            tunnel: w520 -> [w528]
            tunnel: [w526] -> w519
            tunnel: [w525] -> w518
            stop <- w536 stop-if-true
            n205 = global read "Robot Global Data.vi" "Competition Robot?"() -> (w539:bool)
            n206 = call "WPI_SimpleGyro_Get Angle.vi"("SimpleGyroDevRef"=w528) -> ("Angle"=w529:dbl)  [unwired: 8 in, 2 out]
            n207 = call-poly <vilib>:"PID.vi"("output range"=cluster{"output high":dbl, "output low":dbl} {"output high"=0.2, "output low"=-0.2}, "PID gains"=T2 {"proportional gain (Kc)"=1.0, "integral time (Ti, min)"=0.03, "derivative time (Td, min)"=0.005}, "process variable"=w529, "setpoint"=180.0) -> ("output"=w527:dbl)  [unwired: 6 in, 1 out]
            n208 = case shown="False" w539 {
              tunnel: w535 -> [w544 w549]
              tunnel: w527 -> [w543 w547]
              tunnel: [w541 w548] -> w526
              tunnel: [w540 w547] -> w525
              frame True {
                n209 = Multiply(x=w543, y=-1.0) -> (x*y=w540:dbl)
                n210 = call-poly <vilib>:"WPI_RobotDriveHolonomicDrive.vi"("Rotation"=w540, "Y"=0.4 ("X axis value"), "X"=0.0 ("X axis value"), "RobotDriveDevRef"=w544) -> ("RobotDriveDevRef"=w541:T5)  [unwired: 5 in, 2 out]
              }
              frame False {
                n211 = call-poly <vilib>:"WPI_RobotDriveHolonomicDrive.vi"("Rotation"=w547, "Y"=-0.4 ("X axis value"), "X"=0.0 ("X axis value"), "RobotDriveDevRef"=w549) -> ("RobotDriveDevRef"=w548:T5)  [unwired: 5 in, 2 out]
              }
            }
            n212 = call <vilib>:"WPI_EncoderGet.vi"("EncoderDevRef"=w534) -> ("Distance"=w538:dbl, "EncoderDevRef"=w533:T14)  [unwired: 5 in, 4 out]
            n213 = Greater Or Equal?(x=w538, y=1750.0) -> (x >= y?=w536:bool)
          }
        }
        frame #15 {
          w555 = 0.0 ("X")
          n214 = call <vilib>:"WPI_EncoderReset.vi"("EncoderDevRef"=w556) -> ()  [unwired: 9 in, 2 out]
          n215 = call-poly <vilib>:"WPI_RobotDriveHolonomicDrive.vi"("Rotation"=w553, "Y"=w555, "X"=w555, "RobotDriveDevRef"=w554) -> ()  [unwired: 5 in, 3 out]
        }
        frame #16 {
          # "Strafe right"
          n216 = Unbundle By Name(w557) -> ("RobotDriveDevRef"=w559:T5, "EncoderDevRef"=w558:T14)
          n217 = while {
            tunnel: w559 -> [w562]
            tunnel: w558 -> [w561]
            tunnel: [w560] -> _
            stop <- w563 stop-if-true
            n218 = global read "Robot Global Data.vi" "Competition Robot?"() -> (w567:bool)
            n219 = Wait (ms)(milliseconds to wait=u32 30) -> ()  [unwired: 1 out]
            n220 = case shown="False" w567 {
              tunnel: w562 -> [w568 w572]
              frame True {
                n221 = call-poly <vilib>:"WPI_RobotDriveHolonomicDrive.vi"("Rotation"=0.0, "Y"=-1.0 ("X axis value"), "X"=0.0 ("X axis value"), "RobotDriveDevRef"=w568) -> ()  [unwired: 5 in, 3 out]
              }
              frame False {
                n222 = call-poly <vilib>:"WPI_RobotDriveHolonomicDrive.vi"("Rotation"=0.0, "Y"=1.0 ("X axis value"), "X"=0.0 ("X axis value"), "RobotDriveDevRef"=w572) -> ()  [unwired: 5 in, 3 out]
              }
            }
            n223 = call <vilib>:"WPI_EncoderGet.vi"("EncoderDevRef"=w561) -> ("Distance"=w565:dbl, "EncoderDevRef"=w560:T14)  [unwired: 5 in, 4 out]
            n224 = Greater Or Equal?(x=w565, y=-1660.0) -> (x >= y?=w563:bool)
          }
        }
        frame #17 {
          n225 = while {
            tunnel: w578 -> [w588]
            tunnel: [w580] -> w576
            tunnel: [w579] -> w577
            stop <- w585 stop-if-true
            n226 = Unbundle By Name(w588) -> ("MotorControlDevRef"=w587:T6, "MotorControlDevRef"=w586:T6)
            n227 = while {
              tunnel: w587 -> [w599]
              tunnel: [w597] -> w583
              tunnel: [w596] -> w580
              stop <- w597 stop-if-true
              n228 = call "Elapsed Time7"() -> ("Time has Elapsed"=w597:bool)  [unwired: 12 in, 7 out]
              n229 = call <vilib>:"WPI_MotorControlSetOutput.vi"("Output"=1.0, "MotorControlDevRef"=w599) -> ("MotorControlDevRef"=w596:T6)  [unwired: 7 in, 2 out]
            }
            n230 = global read "Robot Global Data.vi" "Competition Robot?"() -> (w584:bool)
            n231 = while {
              tunnel: w586 -> [w595]
              tunnel: w584 -> [w593]
              tunnel: [w590] -> w582
              tunnel: [w589] -> w579
              stop <- w590 stop-if-true
              n232 = Select(t=-1.0, s=w593, f=0.0) -> (s? t:f=w594:dbl)
              n233 = call "ARI Time6"() -> ("Time has Elapsed"=w590:bool)  [unwired: 12 in, 7 out]
              n234 = call <vilib>:"WPI_MotorControlSetOutput.vi"("Output"=w594, "MotorControlDevRef"=w595) -> ("MotorControlDevRef"=w589:T6)  [unwired: 7 in, 2 out]
            }
            n235 = And(x=w582, y=w583) -> (x .and. y?=w581:bool)
            n236 = Select(t=w581, s=w584, f=w583) -> (s? t:f=w585:bool)
          }
        }
        frame #18 {
          n237 = call <vilib>:"WPI_MotorControlSetOutput.vi"("Output"=0.0, "MotorControlDevRef"=w602) -> ()  [unwired: 7 in, 3 out]
          n238 = call <vilib>:"WPI_MotorControlSetOutput.vi"("Output"=0.0, "MotorControlDevRef"=w603) -> ()  [unwired: 7 in, 3 out]
        }
        frame #19 {
          n239 = Unbundle By Name(w605) -> ("SimpleGyroDevRef"=w606:T3, "RobotDriveDevRef"=w607:T5)
          n240 = call "WPI_SimpleGyro_Get Angle.vi"("SimpleGyroDevRef"=w606) -> ("Angle"=w608:dbl)  [unwired: 8 in, 2 out]
          n241 = call-poly <vilib>:"WPI_RobotDriveHolonomicDrive.vi"("Rotation"=0.0, "Gyro Angle"=w608, "Y"=0.0, "X"=0.0, "RobotDriveDevRef"=w607) -> ()  [unwired: 4 in, 3 out]
        }
      }
    }
    frame "Can Left" {
      n242 = call "WPI_SimpleGyro_RefNum Registry Get.vi"("refnum name"="SimpleGyro") -> ("error out"=w627:errorcluster, "SimpleGyroDevRef"=w631:T3)  [unwired: 9 in]
      n243 = call <vilib>:"WPI_RobotDriveRefNum Registry Get.vi"("refnum name"="Four Motors") -> ("error out"=w626:errorcluster, "RobotDriveDevRef"=w630:T5)  [unwired: 1 in, 8 out]
      n244 = call <vilib>:"WPI_EncoderRefNum Registry Get.vi"("refnum name"="Left Front Drive Encoder") -> ("error out"=w625:errorcluster, "EncoderDevRef"=w629:T14)  [unwired: 9 in]
      n245 = call <vilib>:"WPI_MotorControlRefNum Registry Get.vi"("refnum name"="ARI Motor") -> ("error out"=w624:errorcluster, "MotorControlDevRef"=w628:T6)  [unwired: 9 in]
      n246 = call <vilib>:"WPI_RelayRefNum Registry Get.vi"("refnum name"="Clamper Motor") -> ("error out"=w621:errorcluster, "RelayDevRef"=w622:T18)  [unwired: 9 in]
      n247 = Bundle("SimpleGyroDevRef"=w631, "RobotDriveDevRef"=w630, "EncoderDevRef"=w629, "MotorControlDevRef"=w628, "RelayDevRef"=w622) -> (w616:T21)  [unwired: 1 in]
      n248 = Bundle("error out"=w627, "error out"=w626, "error out"=w625, "error out"=w624, "error out"=w621) -> ()  [unwired: 1 in, 1 out]
      n249 = flat-sequence {
        tunnel: [w643] -> w617
        tunnel: w616 -> [w643]
        tunnel: [w648] -> w641
        tunnel: [w647] -> w640
        tunnel: [w646] -> w618
        tunnel: w617 -> [w646]
        tunnel: w641 -> [w656]
        tunnel: w640 -> [w655]
        tunnel: [w654] -> w619
        tunnel: w618 -> [w654]
        tunnel: [w661] -> w639
        tunnel: [w660] -> w638
        tunnel: [w659] -> w620
        tunnel: w619 -> [w659]
        tunnel: w639 -> [w669]
        tunnel: w638 -> [w668]
        tunnel: w620 -> [w667]
        tunnel: [w667] -> w615
        tunnel: [w674] -> w637
        tunnel: [w673] -> w636
        tunnel: w615 -> [w672]
        tunnel: [w671] -> w613
        tunnel: w637 -> [w699]
        tunnel: w636 -> [w698]
        tunnel: [w697] -> w614
        tunnel: w613 -> [w697]
        tunnel: w614 -> [w701]
        tunnel: [w700] -> w612
        tunnel: w612 -> [w722]
        frame #0 {
          n250 = Unbundle By Name(w643) -> ("SimpleGyroDevRef"=w644:T3, "EncoderDevRef"=w642:T14)
          n251 = call "WPI_SimpleGyro_Reset.vi"("SimpleGyroDevRef"=w644) -> ()  [unwired: 9 in, 2 out]
          n252 = call <vilib>:"WPI_EncoderReset.vi"("EncoderDevRef"=w642) -> ()  [unwired: 9 in, 2 out]
        }
        frame #1 {
          n253 = Unbundle By Name(w646) -> ("RelayDevRef"=w645:T18)
          n254 = while {
            tunnel: [w652] -> w648
            tunnel: [w651] -> w647
            tunnel: w645 -> [w649]
            stop <- w650 stop-if-true
            n255 = call "Clamper Time3"() -> ("Time has Elapsed"=w650:bool)  [unwired: 12 in, 7 out]
            n256 = call <vilib>:"WPI_RelaySet.vi"("RelayValue"=WPI_RelayValue."Forward", "RelayDevRef"=w649) -> ("error out"=w651:errorcluster, "RelayDevRef"=w652:T18)  [unwired: 8 in]
          }
        }
        frame #2 {
          n257 = call <vilib>:"WPI_RelaySet.vi"("error in (no error)"=w655, "RelayValue"=WPI_RelayValue."Off", "RelayDevRef"=w656) -> ()  [unwired: 7 in, 2 out]
        }
        frame #3 {
          n258 = Unbundle By Name(w659) -> ("MotorControlDevRef"=w658:T6)
          n259 = while {
            tunnel: [w664] -> w661
            tunnel: [w663] -> w660
            tunnel: w658 -> [w662]
            stop <- w666 stop-if-true
            n260 = call "ARI Time3"() -> ("Time has Elapsed"=w666:bool)  [unwired: 12 in, 7 out]
            n261 = call <vilib>:"WPI_MotorControlSetOutput.vi"("Output"=1.0, "MotorControlDevRef"=w662) -> ("error out"=w664:errorcluster, "MotorControlDevRef"=w663:T6)  [unwired: 7 in, 1 out]
          }
        }
        frame #4 {
          n262 = call <vilib>:"WPI_MotorControlSetOutput.vi"("error in (no error)"=w669, "Output"=0.0, "MotorControlDevRef"=w668) -> ()  [unwired: 6 in, 3 out]
        }
        frame #5 {
          n263 = while {
            tunnel: [w683] -> w674
            tunnel: [w682] -> w673
            tunnel: w672 -> [w678]
            tunnel: [w678] -> w671
            stop <- w684 stop-if-true
            n264 = Unbundle By Name(w678) -> ("EncoderDevRef"=w677:T14, "SimpleGyroDevRef"=w676:T3, "RobotDriveDevRef"=w675:T5)
            n265 = Wait (ms)(milliseconds to wait=u32 30) -> ()  [unwired: 1 out]
            n266 = global read "Robot Global Data.vi" "Competition Robot?"() -> (w680:bool)
            n267 = call <vilib>:"WPI_EncoderGet.vi"("EncoderDevRef"=w677) -> ("error out"=w682:errorcluster, "Distance"=w686:dbl, "EncoderDevRef"=w683:T14)  [unwired: 5 in, 3 out]
            n268 = Greater Or Equal?(x=w686, y=1660.0) -> (x >= y?=w684:bool)
            n269 = call "WPI_SimpleGyro_Get Angle.vi"("SimpleGyroDevRef"=w676) -> ("Angle"=w681:dbl)  [unwired: 8 in, 2 out]
            n270 = case shown="False" w680 {
              tunnel: w681 -> [w688 w693]
              tunnel: w675 -> [w687 w692]
              frame True {
                n271 = call-poly <vilib>:"WPI_RobotDriveHolonomicDrive.vi"("Rotation"=0.0, "Gyro Angle"=w688, "Y"=0.4 ("X axis value"), "X"=0.0 ("X axis value"), "RobotDriveDevRef"=w687) -> ()  [unwired: 4 in, 3 out]
              }
              frame False {
                n272 = call-poly <vilib>:"WPI_RobotDriveHolonomicDrive.vi"("Rotation"=0.0, "Gyro Angle"=w693, "Y"=-0.4 ("X axis value"), "X"=0.0 ("X axis value"), "RobotDriveDevRef"=w692) -> ()  [unwired: 4 in, 3 out]
              }
            }
          }
        }
        frame #6 {
          n273 = call <vilib>:"WPI_EncoderReset.vi"("error in (no error)"=w698, "EncoderDevRef"=w699) -> ()  [unwired: 8 in, 2 out]
        }
        frame #7 {
          n274 = while {
            tunnel: w701 -> [w704]
            tunnel: [w704] -> w700
            stop <- w706 stop-if-true
            n275 = Unbundle By Name(w704) -> ("SimpleGyroDevRef"=w703:T3, "RobotDriveDevRef"=w702:T5)
            n276 = global read "Robot Global Data.vi" "Competition Robot?"() -> (w708:bool)
            n277 = Wait (ms)(milliseconds to wait=u32 30) -> ()  [unwired: 1 out]
            n278 = call "WPI_SimpleGyro_Get Angle.vi"("SimpleGyroDevRef"=w703) -> ("Angle"=w707:dbl)  [unwired: 8 in, 2 out]
            n279 = case shown="True" w708 {
              tunnel: w707 -> [w711 w716]
              tunnel: w702 -> [w710 w715]
              frame True {
                n280 = call-poly <vilib>:"WPI_RobotDriveHolonomicDrive.vi"("Rotation"=0.25, "Gyro Angle"=w711, "Y"=0.0 ("X axis value"), "X"=0.0 ("X axis value"), "RobotDriveDevRef"=w710) -> ()  [unwired: 4 in, 3 out]
              }
              frame False {
                n281 = call-poly <vilib>:"WPI_RobotDriveHolonomicDrive.vi"("Rotation"=-0.5, "Gyro Angle"=w716, "Y"=0.0 ("X axis value"), "X"=0.0 ("X axis value"), "RobotDriveDevRef"=w715) -> ()  [unwired: 4 in, 3 out]
              }
            }
            n282 = Less Or Equal?(x=w707, y=-80.0) -> (x <= y?=w706:bool)
          }
        }
        frame #8 {
          n283 = Unbundle By Name(w722) -> ("SimpleGyroDevRef"=w721:T3, "RobotDriveDevRef"=w720:T5)
          n284 = call "WPI_SimpleGyro_Get Angle.vi"("SimpleGyroDevRef"=w721) -> ("Angle"=w723:dbl)  [unwired: 8 in, 2 out]
          n285 = call-poly <vilib>:"WPI_RobotDriveHolonomicDrive.vi"("Rotation"=0.0, "Gyro Angle"=w723, "Y"=0.0, "X"=0.0, "RobotDriveDevRef"=w720) -> ()  [unwired: 4 in, 3 out]
        }
      }
    }
    frame "Basic" {
      n286 = call "WPI_SimpleGyro_RefNum Registry Get.vi"("refnum name"="SimpleGyro") -> ("error out"=w736:errorcluster, "SimpleGyroDevRef"=w740:T3)  [unwired: 9 in]
      n287 = call <vilib>:"WPI_RobotDriveRefNum Registry Get.vi"("refnum name"="Four Motors") -> ("error out"=w735:errorcluster, "RobotDriveDevRef"=w739:T5)  [unwired: 1 in, 8 out]
      n288 = call <vilib>:"WPI_EncoderRefNum Registry Get.vi"("refnum name"="Left Front Drive Encoder") -> ("error out"=w734:errorcluster, "EncoderDevRef"=w738:T14)  [unwired: 9 in]
      n289 = call <vilib>:"WPI_MotorControlRefNum Registry Get.vi"("refnum name"="ARI Motor") -> ("error out"=w733:errorcluster, "MotorControlDevRef"=w737:T6)  [unwired: 9 in]
      n290 = call <vilib>:"WPI_RelayRefNum Registry Get.vi"("refnum name"="Clamper Motor") -> ("error out"=w730:errorcluster, "RelayDevRef"=w731:T18)  [unwired: 9 in]
      n291 = Bundle("SimpleGyroDevRef"=w740, "RobotDriveDevRef"=w739, "EncoderDevRef"=w738, "MotorControlDevRef"=w737, "RelayDevRef"=w731) -> (w729:T21)  [unwired: 1 in]
      n292 = Bundle("error out"=w736, "error out"=w735, "error out"=w734, "error out"=w733, "error out"=w730) -> ()  [unwired: 1 in, 1 out]
      n293 = flat-sequence {
        tunnel: w729 -> [w747]
        tunnel: [w747] -> w727
        tunnel: [w753] -> w746
        tunnel: [w752] -> w745
        tunnel: [w751] -> w728
        tunnel: w727 -> [w750]
        tunnel: w746 -> [w783]
        tunnel: w745 -> [w782]
        tunnel: w728 -> [w778]
        frame #0 {
          n294 = Unbundle By Name(w747) -> ("SimpleGyroDevRef"=w749:T3, "EncoderDevRef"=w748:T14)
          n295 = call "WPI_SimpleGyro_Reset.vi"("SimpleGyroDevRef"=w749) -> ()  [unwired: 9 in, 2 out]
          n296 = call <vilib>:"WPI_EncoderReset.vi"("EncoderDevRef"=w748) -> ()  [unwired: 9 in, 2 out]
        }
        frame #1 {
          n297 = while {
            tunnel: [w764] -> w753
            tunnel: [w763] -> w752
            tunnel: [w756] -> w751
            tunnel: w750 -> [w755]
            stop <- w765 stop-if-true
            n298 = Unbundle By Name(w755) -> ("EncoderDevRef"=w760:T14, "SimpleGyroDevRef"=w759:T3, "RobotDriveDevRef"=w758:T5)
            n299 = Wait (ms)(milliseconds to wait=u32 30) -> ()  [unwired: 1 out]
            n300 = global read "Robot Global Data.vi" "Competition Robot?"() -> (w762:bool)
            n301 = call "WPI_SimpleGyro_Get Angle.vi"("SimpleGyroDevRef"=w759) -> ("Angle"=w754:dbl)  [unwired: 8 in, 2 out]
            n302 = call "Direction Correction.vi"("Gyro Value"=w754) -> ("Z Value"=w757:dbl)  [unwired: 10 in]
            n303 = call <vilib>:"WPI_EncoderGet.vi"("EncoderDevRef"=w760) -> ("error out"=w763:errorcluster, "Distance"=w767:dbl, "EncoderDevRef"=w764:T14)  [unwired: 5 in, 3 out]
            n304 = case shown="False" w762 {
              tunnel: w758 -> [w770 w774]
              tunnel: w757 -> [w769 _]
              tunnel: [w768 w773] -> w756
              frame True {
                n305 = call-poly <vilib>:"WPI_RobotDriveHolonomicDrive.vi"("Rotation"=w769, "Y"=0.6 ("X axis value"), "X"=0.0 ("X axis value"), "RobotDriveDevRef"=w770) -> ("RobotDriveDevRef"=w768:T5)  [unwired: 5 in, 2 out]
              }
              frame False {
                n306 = call-poly <vilib>:"WPI_RobotDriveHolonomicDrive.vi"("Rotation"=0.0, "Y"=-0.4 ("X axis value"), "X"=0.0 ("X axis value"), "RobotDriveDevRef"=w774) -> ("RobotDriveDevRef"=w773:T5)  [unwired: 5 in, 2 out]
              }
            }
            n307 = Greater Or Equal?(x=w767, y=1660.0) -> (x >= y?=w765:bool)
          }
        }
        frame #2 {
          n308 = while {
            tunnel: w783 -> [w786]
            tunnel: w782 -> [w785]
            stop <- FALSE stop-if-true
            n309 = call <vilib>:"WPI_EncoderReset.vi"("error in (no error)"=w785, "EncoderDevRef"=w786) -> ()  [unwired: 8 in, 2 out]
          }
          n310 = call-poly <vilib>:"WPI_RobotDriveHolonomicDrive.vi"("Rotation"=0.0, "Y"=0.0 ("X axis value"), "X"=0.0 ("X axis value"), "RobotDriveDevRef"=w778) -> ()  [unwired: 5 in, 3 out]
        }
      }
    }
  }
  n311 = while {
    stop <- FALSE stop-if-true
    n312 = Wait (ms)(milliseconds to wait=u32 20) -> ()  [unwired: 1 out]
    n313 = call <vilib>:"WPI_DriverStationReport Robot Code State.vi"("Autonomous"=TRUE) -> ()  [unwired: 10 in, 1 out]
  }
  n314 = disable-structure shown="Disabled" {
    frame Disabled {
      # "go forward for 1 second"
      # "go forward for 1 second"
      n315 = call <vilib>:"WPI_RobotDriveRefNum Registry Get.vi"("refnum name"="Four Motors") -> ("RobotDriveDevRef"=w799:T5)  [unwired: 1 in, 9 out]
      n316 = call-poly <vilib>:"WPI_RobotDriveHolonomicDrive.vi"("Rotation"=0.0, "Y"=0.5 ("X axis value"), "X"=0.0 ("X axis value"), "RobotDriveDevRef"=w799) -> ("Motor Values"=w796:dbl[], "RobotDriveDevRef"=w802:T5)  [unwired: 5 in, 1 out]
      n317 = call <vilib>:"WPI_RobotDriveDelayAndUpdateSafety.vi"("Delay (s)"=4.0, "RobotDriveDevRef"=w802) -> ("RobotDriveDevRef 2"=w790:T5)  [unwired: 8 in, 1 out]
      n318 = call-poly <vilib>:"WPI_RobotDriveHolonomicDrive.vi"("Rotation"=0.0, "Y"=0.0 ("X axis value"), "X"=0.0 ("X axis value"), "RobotDriveDevRef"=w790) -> ("Motor Values"=w791:dbl[])  [unwired: 5 in, 2 out]
      n319 = call-poly <vilib>:"SD Write Value.vi"("Numeric Array"=w791, "Name"="RobotDrive Motors") -> ()  [unwired: 8 in, 2 out]
      n320 = call-poly <vilib>:"SD Write Value.vi"("Numeric Array"=w796, "Name"="RobotDrive Motors") -> ()  [unwired: 8 in, 2 out]
    }
    frame Enabled {
    }
  }
